vi "toJSON.vi"(8 "error in (no error)":errorcluster, 11 "tBSON_I32 in":refnum<class "tBSON_I32.lvclass">) -> (0 "error out":errorcluster, 2 "JSON":string, 3 "tBSON_I32 out":refnum<class "tBSON_I32.lvclass">)   [LabVIEW 2013, in "BSON.lvlib" / "tBSON_I32.lvclass"]
uses:
  tBSON_I32.lvclass
  tBSONElement/tBSONElement.lvclass
  getValue.vi
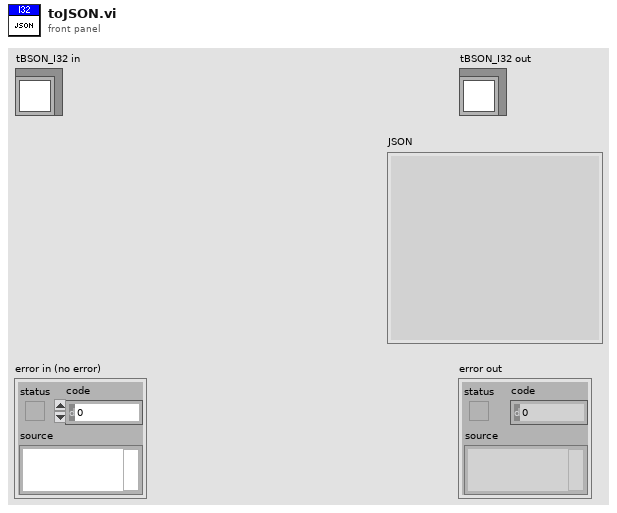
[diagram p1: front panel]
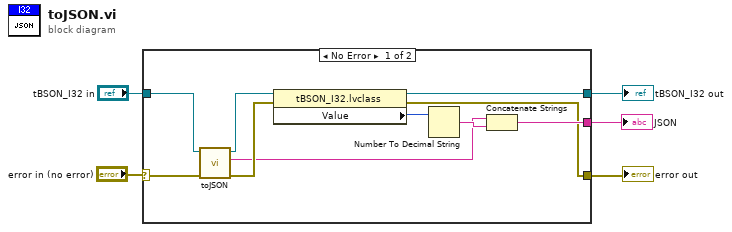
[diagram p0: block diagram]
diagram:
  n1 = case shown="No Error" "error in (no error)" {
    selector: "error in (no error)" -> [w14 w16]
    tunnel: "tBSON_I32 in" -> [w15 w17]
    tunnel: [w9 w16] -> w3
    tunnel: [w8 w17] -> w2
    tunnel: [w10 _] -> w1
    frame No Error {
      n2 = call-parent "toJSON.vi"("error in (no error)"=w14, "tBSONElement in"=w15) -> ("error out"=w12:errorcluster, "JSON"=w6:string, "tBSONElement out"=w13:refnum<class "tBSON_I32.lvclass">)  [unwired: 7 in]
      n3 = property class="tBSON_I32.lvclass"(reference=w13, error in=w12) -> (reference out=w8:refnum<class "tBSON_I32.lvclass">, error out=w9:errorcluster, "Value"=w11:i32)
      n4 = Number To Decimal String(number=w11) -> (decimal integer string=w7:string)  [unwired: 1 in]
      n5 = Concatenate Strings(w6, w7) -> (w10:string)
    }
    frame Error {
    }
  }
  "error out" <- w3
  "tBSON_I32 out" <- w2
  "JSON" <- w1
